vi "CT_CalcPSChargeDelta.vi"(0 "Charge Formation":bool=TRUE, 1 "Form PS Voltage \nSet Point":dbl(slide)=14.5 caption="Form Voltage" min=0.0 max=25.0 step=0.5 scale=0.0..25.0, 2 "Formation PS1 Modules":u8 caption="Formation Modules" max=100, 3 "Charge Acceleration":bool=TRUE, 4 "Acc PS Voltage \nSet Point":dbl(slide)=17.5 caption="Acc Voltage" min=0.0 max=25.0 step=0.5 scale=0.0..25.0, 5 "Acceleration PS2 Modules":u8 max=100, 6 "Acceleration PS3 Modules":u8 max=100) -> (20 "Longest Time":dbl, 21 "Formation PS1 Caps":u8 caption="Formation Caps", 23 "Acceleration PS2 Caps":u8, 24 "First PS Delay":dbl caption="Charge Delta (s) PS1", 26 "Acceleration PS3 Caps":u8, 27 "Second PS Delay":dbl caption="Charge Delta (s) PS2")   [LabVIEW 2009]
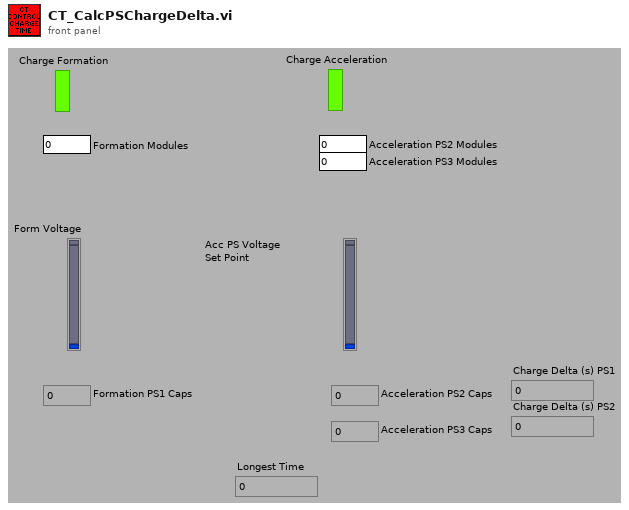
[diagram p1: front panel]
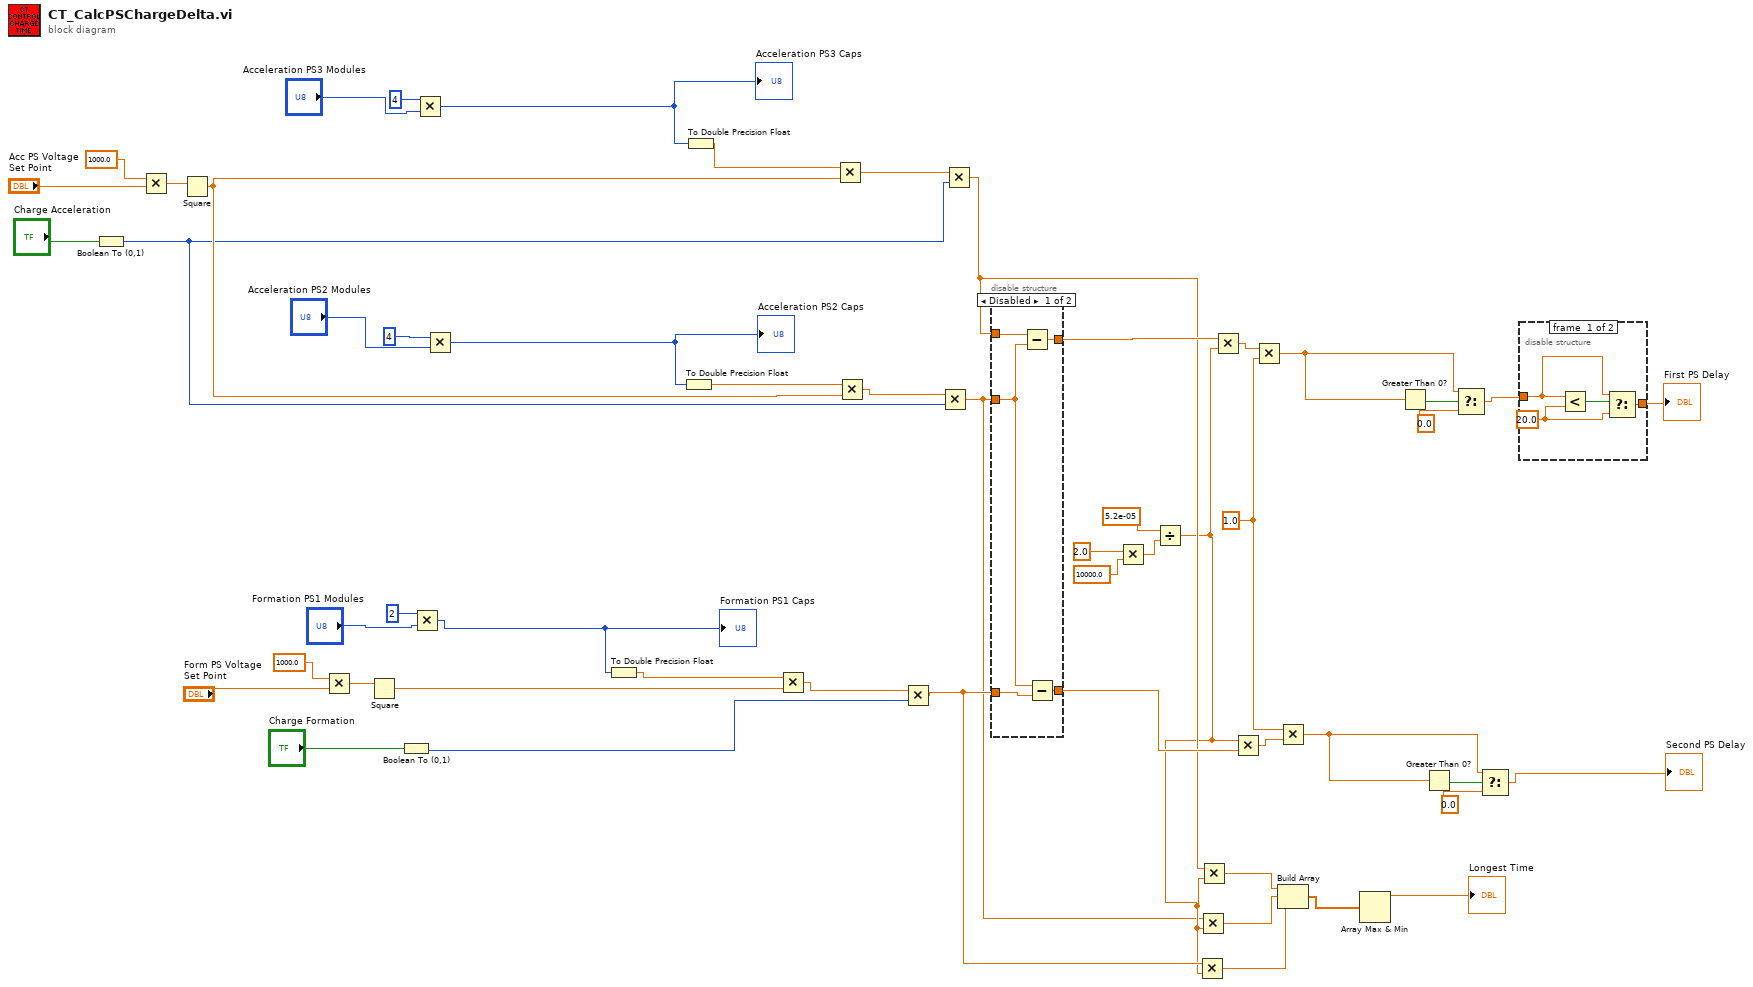
[diagram p0: block diagram]
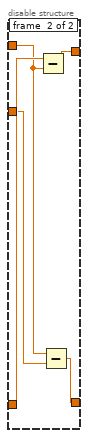
[diagram p2: hidden frame]
diagram:
  w14 = 1.0
  n1 = Boolean To (0,1)(Boolean="Charge Acceleration") -> (0, 1=w27:i16)
  n2 = Multiply(x=1000.0, y="Acc PS Voltage \nSet Point") -> (x*y=w39:dbl)
  n3 = Square(x=w39) -> (x^2=w28:dbl)
  n4 = Multiply(x=1000.0, y="Form PS Voltage \nSet Point") -> (x*y=w35:dbl)
  n5 = Square(x=w35) -> (x^2=w52:dbl)
  n6 = Boolean To (0,1)(Boolean="Charge Formation") -> (0, 1=w50:i16)
  n7 = Multiply(x=2, y="Formation PS1 Modules") -> (x*y=w18:i32)
  "Formation PS1 Caps" <- w18
  n8 = Multiply(x=4, y="Acceleration PS3 Modules") -> (x*y=w10:i32)
  "Acceleration PS3 Caps" <- w10
  n9 = Multiply(x=4, y="Acceleration PS2 Modules") -> (x*y=w13:i32)
  "Acceleration PS2 Caps" <- w13
  n10 = To Double Precision Float(number=w18) -> (double precision float=w16:dbl)
  n11 = To Double Precision Float(number=w13) -> (double precision float=w20:dbl)
  n12 = To Double Precision Float(number=w10) -> (double precision float=w49:dbl)
  n13 = Multiply(x=w16, y=w52) -> (x*y=w51:dbl)
  n14 = Multiply(x=w49, y=w28) -> (x*y=w48:dbl)
  n15 = Multiply(x=w20, y=w28) -> (x*y=w19:dbl)
  n16 = Multiply(x=w51, y=w50) -> (x*y=w8:dbl)
  n17 = Multiply(x=w19, y=w27) -> (x*y=w1:dbl)
  n18 = Multiply(x=w48, y=w27) -> (x*y=w9:dbl)
  n19 = disable-structure shown="Disabled" {
    disable-tunnel: [w59 w63] -> w47
    disable-tunnel: [w58 w60] -> w26
    disable-tunnel: w9 -> [w57 w62]
    disable-tunnel: w8 -> [w56 w64]
    disable-tunnel: w1 -> [w55 w61]
    frame #0 {
      n20 = Subtract(x=w57, y=w55) -> (x-y=w59:dbl)
      n21 = Subtract(x=w55, y=w56) -> (x-y=w58:dbl)
    }
    frame #1 {
      n22 = Subtract(x=w64, y=w62) -> (x-y=w63:dbl)
      n23 = Subtract(x=w62, y=w61) -> (x-y=w60:dbl)
    }
  }
  n24 = Multiply(x=2.0, y=10000.0) -> (x*y=w33:dbl)
  n25 = Divide(x=5.2e-05, y=w33) -> (x/y=w2:dbl)
  n26 = Multiply(x=w8, y=w2) -> (x*y=w5:dbl)
  n27 = Multiply(x=w1, y=w2) -> (x*y=w6:dbl)
  n28 = Multiply(x=w9, y=w2) -> (x*y=w7:dbl)
  n29 = Multiply(x=w47, y=w2) -> (x*y=w15:dbl)
  n30 = Multiply(x=w2, y=w26) -> (x*y=w22:dbl)
  n31 = Multiply(x=w15, y=w14) -> (x*y=w34:dbl)
  n32 = Multiply(x=w14, y=w22) -> (x*y=w23:dbl)
  n33 = Build Array(w7, w6, w5) -> (w4:dbl[])
  n34 = Array Max & Min(array=w4) -> (max value=→"Longest Time":dbl)  [unwired: 3 out]
  n35 = Greater Than 0?(x=w34) -> (x > 0?=w46:bool)
  n36 = Greater Than 0?(x=w23) -> (x > 0?=w25:bool)
  n37 = Select(t=w34, s=w46, f=0.0) -> (s? t:f=w44:dbl)
  n38 = Select(t=w23, s=w25, f=0.0) -> (s? t:f=→"Second PS Delay":dbl)
  n39 = disable-structure shown="Enabled" {
    disable-tunnel: w44 -> [w65 w69]
    disable-tunnel: [w66 w69] -> w41
    frame #0 {
      w67 = 20.0
      n40 = Less?(x=w65, y=w67) -> (x < y?=w68:bool)
      n41 = Select(t=w65, s=w68, f=w67) -> (s? t:f=w66:dbl)
    }
    frame #1 {
    }
  }
  "First PS Delay" <- w41
